vi "PicoScopeospaExampleBlock.vi"() -> ()   [LabVIEW 2010]
uses:
  shared/PicoBuffers.ctl
  <vilib>/Waveform/DWDTOps.llb/DWDT Analog to Digital.vi
  PicoScopepsospaLib/PicoScopeospaDigitalChannelSettings.ctl
  PicoScopepsospaLib/PicoScopeospaAnalogChannelSettings.ctl
  shared/Acquisition Settings.ctl
  shared/Buffer and Transfer Settings.ctl
panel:
  in  "timeIntervalRequested":dbl=2e-10 format="%#6_6p"
  in  "Write ChA to TDMS":bool
  in  "Channels":T1={"Channel A Settings "={"Enabled"=TRUE, "Coupling"=1, "Range"=8, "Analogue Offset"=0.0, "BandWidth"=0, "PROBE_RANGE_INFO"=1}, "Channel B Settings "={"Enabled"=FALSE, "Coupling"=1, "Range"=8, "Analogue Offset"=0.0, "BandWidth"=0, "PROBE_RANGE_INFO"=1}, "Channel C Settings "={"Enabled"=FALSE, "Coupling"=1, "Range"=8, "Analogue Offset"=0.0, "BandWidth"=0, "PROBE_RANGE_INFO"=1}, "Channel D Settings "={"Enabled"=FALSE, "Coupling"=1, "Range"=8, "Analogue Offset"=0.0, "BandWidth"=0, "PROBE_RANGE_INFO"=1}, "Channel E Settings "={"Enabled"=FALSE, "Coupling"=50, "Range"=5, "Analogue Offset"=0.0, "BandWidth"=0, "PROBE_RANGE_INFO"=0}, "Channel F Settings "={"Enabled"=FALSE, "Coupling"=50, "Range"=5, "Analogue Offset"=0.0, "BandWidth"=0, "PROBE_RANGE_INFO"=0}, "Channel G Settings "={"Enabled"=FALSE, "Coupling"=50, "Range"=5, "Analogue Offset"=0.0, "BandWidth"=0, "PROBE_RANGE_INFO"=0}, "Channel H Settings "={"Enabled"=FALSE, "Coupling"=50, "Range"=5, "Analogue Offset"=0.0, "BandWidth"=0, "PROBE_RANGE_INFO"=0}} {"Channel H Settings"."PROBE_RANGE_INFO" items=["PROBE_NONE_NV"=0, "X1_PROBE_NV"=1, "X10_PROBE_NV"=10]; "Channel H Settings"."BandWidth" items=["Full"=0, "100kHz"=100000, "20kHz"=200000, "1MHz"=1000000, "20MHz"=20000000, "25MHz"=25000000, "50MHz"=50000000, "200MHz"=200000000, "250MHz"=250000000, "500MHz"=500000000]; "Channel H Settings"."Range" items=["10mV"=0, "20mV"=1, "50mV"=2, "100mV"=3, "200mV"=4, "500mV"=5, "1V"=6, "2V"=7, "5V"=8, "10V"=9, "20V"=10, "50V"=11, "100V"=12, "200V"=13, "x10_Probe_100mV"=32, "x10_Probe_200mV"=33, "x10_Probe_500mV"=34, "x10_Probe_1V"=35, "x10_Probe_2V"=36, "x10_Probe_5V"=37, "x10_Probe_10V"=38, "x10_Probe_20V"=39, "x10_Probe_50V"=40, "x10_Probe_100V"=41, "x10_Probe_200V"=42, "x10_Probe_500V"=43, "CURRENT_CLAMP_60A_2A"=10500, "CURRENT_CLAMP_60A_5A"=10501, "CURRENT_CLAMP_60A_10A"=10502, "CURRENT_CLAMP_60A_20A"=10503, "CURRENT_CLAMP_60A_50A"=10504, "CURRENT_CLAMP_60A_60A"=10505, "CURRENT_CLAMP_60A_V2_0_5A"=10600, "CURRENT_CLAMP_60A_V2_1A"=10601, "CURRENT_CLAMP_60A_V2_2A"=10602, "CURRENT_CLAMP_60A_V2_5A"=10603, "CURRENT_CLAMP_60A_V2_10A"=10604, "CURRENT_CLAMP_60A_V2_20A"=10605, "CURRENT_CLAMP_60A_V2_50A"=10606, "CURRENT_CLAMP_60A_V2_60A"=10607, "RESISTANCE_LEAD_NEG5_TO_20OHM"=7000, "RESISTANCE_LEAD_NEG50_TO_200OHM"=7001, "RESISTANCE_LEAD_NEG500_TO_2KOHM"=7002, "RESISTANCE_LEAD_NEG5K_TO_20KOHM"=7003, "RESISTANCE_LEAD_NEG50K_TO_LEAD_200KOHM"=7004, "RESISTANCE_LEAD_NEG500K_TO_LEAD_2MOHM"=7005, "RESISTANCE_LEAD_DIODE_TEST"=7006, "HT_NEG3_TO_5KV"=8950, "HT_NEG3_TO_10KV"=8951, "HT_NEG5_TO_20KV"=8952, "HT_NEG5_TO_50KV"=8953, "HT_NEG5_TO_100KV"=8954, "HT_NEG3_TO_5KV_INVERTED"=8955, "HT_NEG3_TO_10KV_INVERTED"=8956, "HT_NEG5_TO_20KV_INVERTED"=8957, "HT_NEG5_TO_50KV_INVERTED"=8958, "HT_NEG5_TO_100KV_INVERTED"=8959, "TEMPERATURE_NEG50_TO_150DEGC"=9000, "PRESSURE_SENSOR_-100k-150k_PASCALS"=9100, "PRESSURE_SENSOR_-100k_TO_400k_PASCALS"=9101, "PRESSURE_SENSOR_-200k_TO_800k_PASCALS"=9102, "PRESSURE_SENSOR_-400k_TO_1600k_PASCALS"=9103, "PRESSURE_SENSOR_-400k_TO_3400k_PASCALS"=9104, "PRESSURE_SENSOR_-150k_TO_1350k_PASCALS"=9105]; "Channel H Settings"."Coupling" items=["AC"=0, "DC 1M Ohm"=1, "DC 50 Ohm"=50]; "Channel G Settings"."PROBE_RANGE_INFO" items=["PROBE_NONE_NV"=0, "X1_PROBE_NV"=1, "X10_PROBE_NV"=10]; "Channel G Settings"."BandWidth" items=["Full"=0, "100kHz"=100000, "20kHz"=200000, "1MHz"=1000000, "20MHz"=20000000, "25MHz"=25000000, "50MHz"=50000000, "200MHz"=200000000, "250MHz"=250000000, "500MHz"=500000000]; "Channel G Settings"."Range" items=["10mV"=0, "20mV"=1, "50mV"=2, "100mV"=3, "200mV"=4, "500mV"=5, "1V"=6, "2V"=7, "5V"=8, "10V"=9, "20V"=10, "50V"=11, "100V"=12, "200V"=13, "x10_Probe_100mV"=32, "x10_Probe_200mV"=33, "x10_Probe_500mV"=34, "x10_Probe_1V"=35, "x10_Probe_2V"=36, "x10_Probe_5V"=37, "x10_Probe_10V"=38, "x10_Probe_20V"=39, "x10_Probe_50V"=40, "x10_Probe_100V"=41, "x10_Probe_200V"=42, "x10_Probe_500V"=43, "CURRENT_CLAMP_60A_2A"=10500, "CURRENT_CLAMP_60A_5A"=10501, "CURRENT_CLAMP_60A_10A"=10502, "CURRENT_CLAMP_60A_20A"=10503, "CURRENT_CLAMP_60A_50A"=10504, "CURRENT_CLAMP_60A_60A"=10505, "CURRENT_CLAMP_60A_V2_0_5A"=10600, "CURRENT_CLAMP_60A_V2_1A"=10601, "CURRENT_CLAMP_60A_V2_2A"=10602, "CURRENT_CLAMP_60A_V2_5A"=10603, "CURRENT_CLAMP_60A_V2_10A"=10604, "CURRENT_CLAMP_60A_V2_20A"=10605, "CURRENT_CLAMP_60A_V2_50A"=10606, "CURRENT_CLAMP_60A_V2_60A"=10607, "RESISTANCE_LEAD_NEG5_TO_20OHM"=7000, "RESISTANCE_LEAD_NEG50_TO_200OHM"=7001, "RESISTANCE_LEAD_NEG500_TO_2KOHM"=7002, "RESISTANCE_LEAD_NEG5K_TO_20KOHM"=7003, "RESISTANCE_LEAD_NEG50K_TO_LEAD_200KOHM"=7004, "RESISTANCE_LEAD_NEG500K_TO_LEAD_2MOHM"=7005, "RESISTANCE_LEAD_DIODE_TEST"=7006, "HT_NEG3_TO_5KV"=8950, "HT_NEG3_TO_10KV"=8951, "HT_NEG5_TO_20KV"=8952, "HT_NEG5_TO_50KV"=8953, "HT_NEG5_TO_100KV"=8954, "HT_NEG3_TO_5KV_INVERTED"=8955, "HT_NEG3_TO_10KV_INVERTED"=8956, "HT_NEG5_TO_20KV_INVERTED"=8957, "HT_NEG5_TO_50KV_INVERTED"=8958, "HT_NEG5_TO_100KV_INVERTED"=8959, "TEMPERATURE_NEG50_TO_150DEGC"=9000, "PRESSURE_SENSOR_-100k-150k_PASCALS"=9100, "PRESSURE_SENSOR_-100k_TO_400k_PASCALS"=9101, "PRESSURE_SENSOR_-200k_TO_800k_PASCALS"=9102, "PRESSURE_SENSOR_-400k_TO_1600k_PASCALS"=9103, "PRESSURE_SENSOR_-400k_TO_3400k_PASCALS"=9104, "PRESSURE_SENSOR_-150k_TO_1350k_PASCALS"=9105]; "Channel G Settings"."Coupling" items=["AC"=0, "DC 1M Ohm"=1, "DC 50 Ohm"=50]; "Channel F Settings"."PROBE_RANGE_INFO" items=["PROBE_NONE_NV"=0, "X1_PROBE_NV"=1, "X10_PROBE_NV"=10]; "Channel F Settings"."BandWidth" items=["Full"=0, "100kHz"=100000, "20kHz"=200000, "1MHz"=1000000, "20MHz"=20000000, "25MHz"=25000000, "50MHz"=50000000, "200MHz"=200000000, "250MHz"=250000000, "500MHz"=500000000]; "Channel F Settings"."Range" items=["10mV"=0, "20mV"=1, "50mV"=2, "100mV"=3, "200mV"=4, "500mV"=5, "1V"=6, "2V"=7, "5V"=8, "10V"=9, "20V"=10, "50V"=11, "100V"=12, "200V"=13, "x10_Probe_100mV"=32, "x10_Probe_200mV"=33, "x10_Probe_500mV"=34, "x10_Probe_1V"=35, "x10_Probe_2V"=36, "x10_Probe_5V"=37, "x10_Probe_10V"=38, "x10_Probe_20V"=39, "x10_Probe_50V"=40, "x10_Probe_100V"=41, "x10_Probe_200V"=42, "x10_Probe_500V"=43, "CURRENT_CLAMP_60A_2A"=10500, "CURRENT_CLAMP_60A_5A"=10501, "CURRENT_CLAMP_60A_10A"=10502, "CURRENT_CLAMP_60A_20A"=10503, "CURRENT_CLAMP_60A_50A"=10504, "CURRENT_CLAMP_60A_60A"=10505, "CURRENT_CLAMP_60A_V2_0_5A"=10600, "CURRENT_CLAMP_60A_V2_1A"=10601, "CURRENT_CLAMP_60A_V2_2A"=10602, "CURRENT_CLAMP_60A_V2_5A"=10603, "CURRENT_CLAMP_60A_V2_10A"=10604, "CURRENT_CLAMP_60A_V2_20A"=10605, "CURRENT_CLAMP_60A_V2_50A"=10606, "CURRENT_CLAMP_60A_V2_60A"=10607, "RESISTANCE_LEAD_NEG5_TO_20OHM"=7000, "RESISTANCE_LEAD_NEG50_TO_200OHM"=7001, "RESISTANCE_LEAD_NEG500_TO_2KOHM"=7002, "RESISTANCE_LEAD_NEG5K_TO_20KOHM"=7003, "RESISTANCE_LEAD_NEG50K_TO_LEAD_200KOHM"=7004, "RESISTANCE_LEAD_NEG500K_TO_LEAD_2MOHM"=7005, "RESISTANCE_LEAD_DIODE_TEST"=7006, "HT_NEG3_TO_5KV"=8950, "HT_NEG3_TO_10KV"=8951, "HT_NEG5_TO_20KV"=8952, "HT_NEG5_TO_50KV"=8953, "HT_NEG5_TO_100KV"=8954, "HT_NEG3_TO_5KV_INVERTED"=8955, "HT_NEG3_TO_10KV_INVERTED"=8956, "HT_NEG5_TO_20KV_INVERTED"=8957, "HT_NEG5_TO_50KV_INVERTED"=8958, "HT_NEG5_TO_100KV_INVERTED"=8959, "TEMPERATURE_NEG50_TO_150DEGC"=9000, "PRESSURE_SENSOR_-100k-150k_PASCALS"=9100, "PRESSURE_SENSOR_-100k_TO_400k_PASCALS"=9101, "PRESSURE_SENSOR_-200k_TO_800k_PASCALS"=9102, "PRESSURE_SENSOR_-400k_TO_1600k_PASCALS"=9103, "PRESSURE_SENSOR_-400k_TO_3400k_PASCALS"=9104, "PRESSURE_SENSOR_-150k_TO_1350k_PASCALS"=9105]; "Channel F Settings"."Coupling" items=["AC"=0, "DC 1M Ohm"=1, "DC 50 Ohm"=50]; "Channel E Settings"."PROBE_RANGE_INFO" items=["PROBE_NONE_NV"=0, "X1_PROBE_NV"=1, "X10_PROBE_NV"=10]; "Channel E Settings"."BandWidth" items=["Full"=0, "100kHz"=100000, "20kHz"=200000, "1MHz"=1000000, "20MHz"=20000000, "25MHz"=25000000, "50MHz"=50000000, "200MHz"=200000000, "250MHz"=250000000, "500MHz"=500000000]; "Channel E Settings"."Range" items=["10mV"=0, "20mV"=1, "50mV"=2, "100mV"=3, "200mV"=4, "500mV"=5, "1V"=6, "2V"=7, "5V"=8, "10V"=9, "20V"=10, "50V"=11, "100V"=12, "200V"=13, "x10_Probe_100mV"=32, "x10_Probe_200mV"=33, "x10_Probe_500mV"=34, "x10_Probe_1V"=35, "x10_Probe_2V"=36, "x10_Probe_5V"=37, "x10_Probe_10V"=38, "x10_Probe_20V"=39, "x10_Probe_50V"=40, "x10_Probe_100V"=41, "x10_Probe_200V"=42, "x10_Probe_500V"=43, "CURRENT_CLAMP_60A_2A"=10500, "CURRENT_CLAMP_60A_5A"=10501, "CURRENT_CLAMP_60A_10A"=10502, "CURRENT_CLAMP_60A_20A"=10503, "CURRENT_CLAMP_60A_50A"=10504, "CURRENT_CLAMP_60A_60A"=10505, "CURRENT_CLAMP_60A_V2_0_5A"=10600, "CURRENT_CLAMP_60A_V2_1A"=10601, "CURRENT_CLAMP_60A_V2_2A"=10602, "CURRENT_CLAMP_60A_V2_5A"=10603, "CURRENT_CLAMP_60A_V2_10A"=10604, "CURRENT_CLAMP_60A_V2_20A"=10605, "CURRENT_CLAMP_60A_V2_50A"=10606, "CURRENT_CLAMP_60A_V2_60A"=10607, "RESISTANCE_LEAD_NEG5_TO_20OHM"=7000, "RESISTANCE_LEAD_NEG50_TO_200OHM"=7001, "RESISTANCE_LEAD_NEG500_TO_2KOHM"=7002, "RESISTANCE_LEAD_NEG5K_TO_20KOHM"=7003, "RESISTANCE_LEAD_NEG50K_TO_LEAD_200KOHM"=7004, "RESISTANCE_LEAD_NEG500K_TO_LEAD_2MOHM"=7005, "RESISTANCE_LEAD_DIODE_TEST"=7006, "HT_NEG3_TO_5KV"=8950, "HT_NEG3_TO_10KV"=8951, "HT_NEG5_TO_20KV"=8952, "HT_NEG5_TO_50KV"=8953, "HT_NEG5_TO_100KV"=8954, "HT_NEG3_TO_5KV_INVERTED"=8955, "HT_NEG3_TO_10KV_INVERTED"=8956, "HT_NEG5_TO_20KV_INVERTED"=8957, "HT_NEG5_TO_50KV_INVERTED"=8958, "HT_NEG5_TO_100KV_INVERTED"=8959, "TEMPERATURE_NEG50_TO_150DEGC"=9000, "PRESSURE_SENSOR_-100k-150k_PASCALS"=9100, "PRESSURE_SENSOR_-100k_TO_400k_PASCALS"=9101, "PRESSURE_SENSOR_-200k_TO_800k_PASCALS"=9102, "PRESSURE_SENSOR_-400k_TO_1600k_PASCALS"=9103, "PRESSURE_SENSOR_-400k_TO_3400k_PASCALS"=9104, "PRESSURE_SENSOR_-150k_TO_1350k_PASCALS"=9105]; "Channel E Settings"."Coupling" items=["AC"=0, "DC 1M Ohm"=1, "DC 50 Ohm"=50]; "Channel D Settings"."BandWidth" items=["Full"=0, "100kHz"=100000, "20kHz"=200000, "1MHz"=1000000, "20MHz"=20000000, "25MHz"=25000000, "50MHz"=50000000, "100MHz"=100000000, "200MHz"=200000000, "250MHz"=250000000, "350MHz"=350000000, "500MHz"=500000000]; "Channel D Settings"."PROBE_RANGE_INFO" items=["PROBE_NONE_NV"=0, "X1_PROBE_NV"=1, "X10_PROBE_NV"=10]; "Channel D Settings"."Range" items=["10mV", "20mV", "50mV", "100mV", "200mV", "500mV", "1V", "2V", "5V", "10V", "20V", "50V", "100V", "200V"]; "Channel D Settings"."Coupling" items=["AC"=0, "DC 1M Ohm"=1, "DC 50 Ohm"=50]; "Channel C Settings"."BandWidth" items=["Full"=0, "100kHz"=100000, "20kHz"=200000, "1MHz"=1000000, "20MHz"=20000000, "25MHz"=25000000, "50MHz"=50000000, "100MHz"=100000000, "200MHz"=200000000, "250MHz"=250000000, "350MHz"=350000000, "500MHz"=500000000]; "Channel C Settings"."PROBE_RANGE_INFO" items=["PROBE_NONE_NV"=0, "X1_PROBE_NV"=1, "X10_PROBE_NV"=10]; "Channel C Settings"."Range" items=["10mV", "20mV", "50mV", "100mV", "200mV", "500mV", "1V", "2V", "5V", "10V", "20V", "50V", "100V", "200V"]; "Channel C Settings"."Coupling" items=["AC"=0, "DC 1M Ohm"=1, "DC 50 Ohm"=50]; "Channel B Settings"."BandWidth" items=["Full"=0, "100kHz"=100000, "20kHz"=200000, "1MHz"=1000000, "20MHz"=20000000, "25MHz"=25000000, "50MHz"=50000000, "100MHz"=100000000, "200MHz"=200000000, "250MHz"=250000000, "350MHz"=350000000, "500MHz"=500000000]; "Channel B Settings"."PROBE_RANGE_INFO" items=["PROBE_NONE_NV"=0, "X1_PROBE_NV"=1, "X10_PROBE_NV"=10]; "Channel B Settings"."Range" items=["10mV", "20mV", "50mV", "100mV", "200mV", "500mV", "1V", "2V", "5V", "10V", "20V", "50V", "100V", "200V"]; "Channel B Settings"."Coupling" items=["AC"=0, "DC 1M Ohm"=1, "DC 50 Ohm"=50]; "Channel A Settings"."PROBE_RANGE_INFO" items=["PROBE_NONE_NV"=0, "X1_PROBE_NV"=1, "X10_PROBE_NV"=10]; "Channel A Settings"."Range" items=["10mV", "20mV", "50mV", "100mV", "200mV", "500mV", "1V", "2V", "5V", "10V", "20V", "50V", "100V", "200V"]; "Channel A Settings"."BandWidth" items=["Full"=0, "100kHz"=100000, "20kHz"=200000, "1MHz"=1000000, "20MHz"=20000000, "25MHz"=25000000, "50MHz"=50000000, "100MHz"=100000000, "200MHz"=200000000, "250MHz"=250000000, "350MHz"=350000000, "500MHz"=500000000]; "Channel A Settings"."Coupling" items=["AC"=0, "DC 1M Ohm"=1, "DC 50 Ohm"=50]}
  out "error out":errorcluster
  in  "Data file":path=path "PicoScopeospaExampleBlock ChA Data"
  out "overflow":i16 format="%010b"
  in  "Apply Settings":bool
  in  "Digital Channels":T2={"Port 0 Settings "={"Enabled"=FALSE, "Threshold Level (Volts)"=1.0}, "Port 1 Settings"={"Enabled"=FALSE, "Threshold Level (Volts)"=1.0}} {"Port 1 Settings"."Threshold Level (Volts)" format="%#_4p"; "Port 0 Settings"."Threshold Level (Volts)" format="%#_4p"}
  in  "Trigger Settings":T3={"Trigger Enabled"=FALSE, "Trigger Threshold (Volts)"=0.0, "Trigger Direction"=2, "Trigger Delay (samples)"=0, "Auto Trigger Time (us)"=1000000, "Trigger Source"=0} {"Trigger Source" items=["Channel A"=0, "Channel B"=1, "Channel C"=2, "Channel D"=3, "Channel E"=4, "Channel F"=5, "Channel G"=6, "Channel H"=7, "Port 0"=128, "Port 1"=129, "Trigger AUX"=1001]; "Auto Trigger Time (us)" format="%.4p"; "Trigger Direction" items=["Above", "Below", "Rising", "Falling", "Rising or Falling"]; "Trigger Threshold (Volts)" format="%#_6p"}
  in  "Buffer and Transfer Settings":T4={"startIndex"=0, "Samples"=10000000, "Down Sample Ratio"=16, "Down-Sample Mode"=2} {"Down-Sample Mode" items=["RAW none"=2147483648, "None"=0, "Aggregate"=1, "Decimate"=2, "Average"=4]; "Down Sample Ratio" step=1; "Samples" format="%_6p"}
  in  "Acquisition Settings":T5={"preTriggerSamples"=0, "postTriggerSamples"=100000000, "timebase"=2} {"postTriggerSamples" format="%_6p"; "preTriggerSamples" format="%_6p"}
  out "Properties Panel":T6 {"Max Total Capture Time Available (sec)" format="%.3p"; "Sample Frequency" format="%.6p"; "Sample Rate" format="%.3p"; "Max Samples Available" format="%_6p"; "Total Capture Time (sec)" format="%.3p"}
  out "Port 0":digitalwaveform(graph)={"t0"=timestamp(0 s since 1904-01-01), "dt"=4e-09, "Y"={"transitions"=[], "data"=[]}}
  in  "stop":bool
  out "Analog Channels":cluster{i32, dbl, "Data":dbl[]}[](graph)
  out "Device Info":T7={"PICO_DRIVER_VERSION"="", "PICO_USB_VERSION"="", "PICO_HARDWARE_VERSION"="", "PICO_VARIANT_INFO"="", "PICO_BATCH_AND_SERIAL"="", "PICO_CAL_DATE"="", "PICO_KERNEL_VERSION"="", "PICO_DIGITAL_HARDWARE_VERSION"="", "PICO_ANALOGUE_HARDWARE_VERSION"="", "PICO_FIRMWARE_VERSION_1"="", "PICO_FIRMWARE_VERSION_2"="", "PICO_IPP_VERSION"="", "PICO_DRIVER_PATH"="", "PICO_FIRMWARE_VERSION_3"="", "PICO_FRONT_PANEL_FIRMWARE_VERSION"="", "Number of Channels"=4, "MSO"=FALSE}
  out "Pico psospa Units":string
  in  "Resolution":u32(ring) items=["8-bit"=0, "12-bit"=1, "14-bit"=2, "15-bit"=3, "16-bit"=4, "10-bit"=10]
  in  "Serial Number":string
  in  "Use Serial Number":bool
  in  "error in (no error)":errorcluster
  # "D8-D15"
  # "DO-D7"
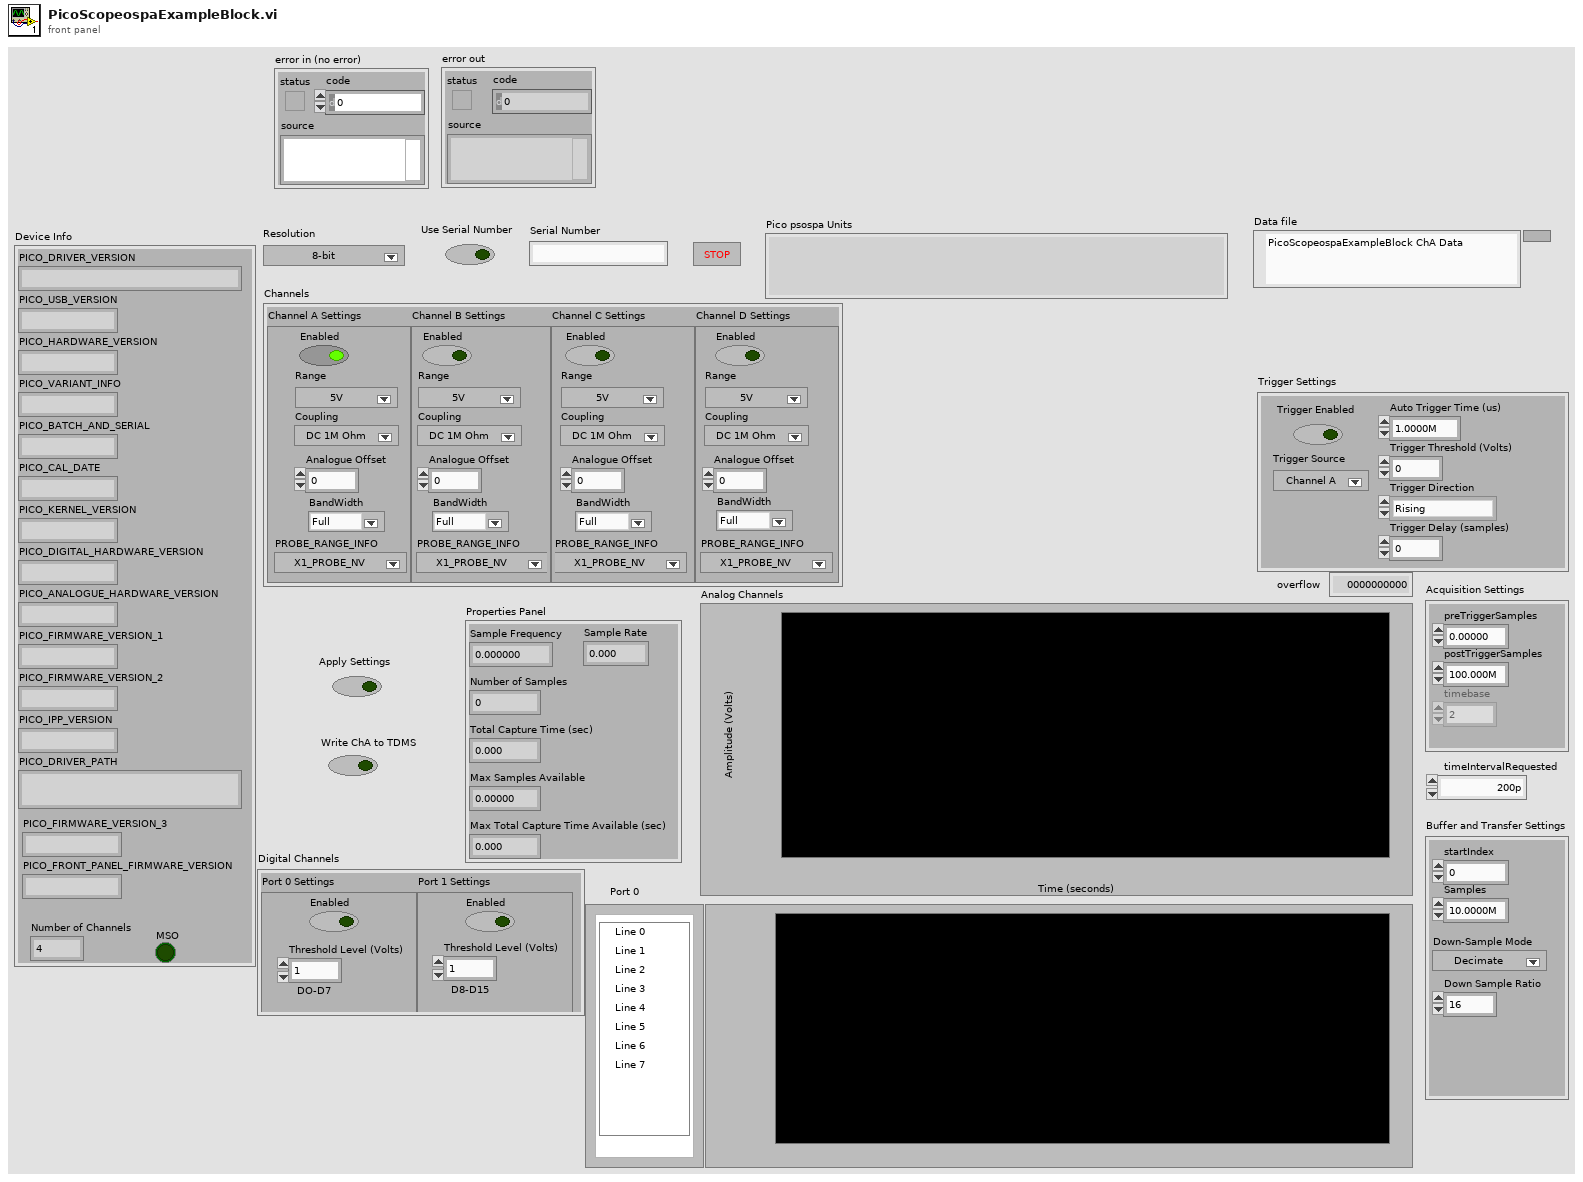
[diagram p1: front panel]
types:
  T1 = typedef "PicoScopeospaAnalogChannelSettings.ctl" = cluster{"Channel A Settings ":cluster{"Enabled":bool, "Coupling":i16, "Range":u16, "Analogue Offset":dbl, "BandWidth":u32, "PROBE_RANGE_INFO":u32}, "Channel B Settings ":cluster{"Enabled":bool, "Coupling":i16, "Range":u16, "Analogue Offset":dbl, "BandWidth":u32, "PROBE_RANGE_INFO":u32}, "Channel C Settings ":cluster{"Enabled":bool, "Coupling":i16, "Range":u16, "Analogue Offset":dbl, "BandWidth":u32, "PROBE_RANGE_INFO":u32}, "Channel D Settings ":cluster{"Enabled":bool, "Coupling":i16, "Range":u16, "Analogue Offset":dbl, "BandWidth":u32, "PROBE_RANGE_INFO":u32}, "Channel E Settings ":cluster{"Enabled":bool, "Coupling":i16, "Range":u16, "Analogue Offset":dbl, "BandWidth":u32, "PROBE_RANGE_INFO":u32}, "Channel F Settings ":cluster{"Enabled":bool, "Coupling":i16, "Range":u16, "Analogue Offset":dbl, "BandWidth":u32, "PROBE_RANGE_INFO":u32}, "Channel G Settings ":cluster{"Enabled":bool, "Coupling":i16, "Range":u16, "Analogue Offset":dbl, "BandWidth":u32, "PROBE_RANGE_INFO":u32}, "Channel H Settings ":cluster{"Enabled":bool, "Coupling":i16, "Range":u16, "Analogue Offset":dbl, "BandWidth":u32, "PROBE_RANGE_INFO":u32}}
  T2 = typedef "PicoScopeospaDigitalChannelSettings.ctl" = cluster{"Port 0 Settings ":cluster{"Enabled":bool, "Threshold Level (Volts)":dbl}, "Port 1 Settings":cluster{"Enabled":bool, "Threshold Level (Volts)":dbl}}
  T3 = cluster{"Trigger Enabled":bool, "Trigger Threshold (Volts)":dbl, "Trigger Direction":u16, "Trigger Delay (samples)":u64, "Auto Trigger Time (us)":u32, "Trigger Source":u32}
  T4 = typedef "Buffer and Transfer Settings.ctl" = cluster{"startIndex":u64, "Samples":u64, "Down Sample Ratio":u64, "Down-Sample Mode":u32}
  T5 = typedef "Acquisition Settings.ctl" = cluster{"preTriggerSamples":u64, "postTriggerSamples":u64, "timebase":u32}
  T6 = cluster{"Sample Frequency":dbl, "Sample Rate":dbl, "Max Samples Available":u64, "Number of Samples":u64, "Total Capture Time (sec) ":dbl, "Max Total Capture Time Available (sec)":dbl}
  T7 = cluster{"PICO_DRIVER_VERSION":string, "PICO_USB_VERSION":string, "PICO_HARDWARE_VERSION":string, "PICO_VARIANT_INFO":string, "PICO_BATCH_AND_SERIAL":string, "PICO_CAL_DATE":string, "PICO_KERNEL_VERSION":string, "PICO_DIGITAL_HARDWARE_VERSION":string, "PICO_ANALOGUE_HARDWARE_VERSION":string, "PICO_FIRMWARE_VERSION_1":string, "PICO_FIRMWARE_VERSION_2":string, "PICO_IPP_VERSION":string, "PICO_DRIVER_PATH":string, "PICO_FIRMWARE_VERSION_3":string, "PICO_FRONT_PANEL_FIRMWARE_VERSION":string, "Number of Channels":i16, "MSO":bool}
  T8 = enum16{"open", "open or create", "create or replace", "create", "open (read-only)"}
  T9 = typedef "PicoBuffers.ctl" = cluster{"Max Buffer Pointers":u64[][][], "Min Buffer Pointers":u64[][][], "StreamingDataInfo":cluster{"Channel":u32, "Down-Sample Mode":u32, "PICO_DATA_TYPE":enum32{"PICO_INT8_T", "PICO_INT16_T", "PICO_INT32_T", "PICO_UINT32_T", "PICO_INT64_T", ""}, "Samples":i32, "bufferIndex":u64, "startIndex":i32, "overflow":i16}[][]}
  T10 = cluster{"Channel A Buffer":i16[], "Channel B Buffer":i16[], "Channel C Buffer":i16[], "Channel D Buffer":i16[], "Channel E Buffer":i16[], "Channel F Buffer":i16[], "Channel G Buffer":i16[], "Channel H Buffer":i16[], "Port 0 Buffer":i16[], "Port 1 Buffer":i16[]}[]
  T11 = cluster{"Channel A Buffer":i16[], "Channel B Buffer":i16[], "Channel C Buffer":i16[], "Channel D Buffer":i16[], "Channel E Buffer":i16[], "Channel F Buffer":i16[], "Channel G Buffer":i16[], "Channel H Buffer":i16[], "Port 0 Buffer":i16[], "Port 1 Buffer":i16[]}
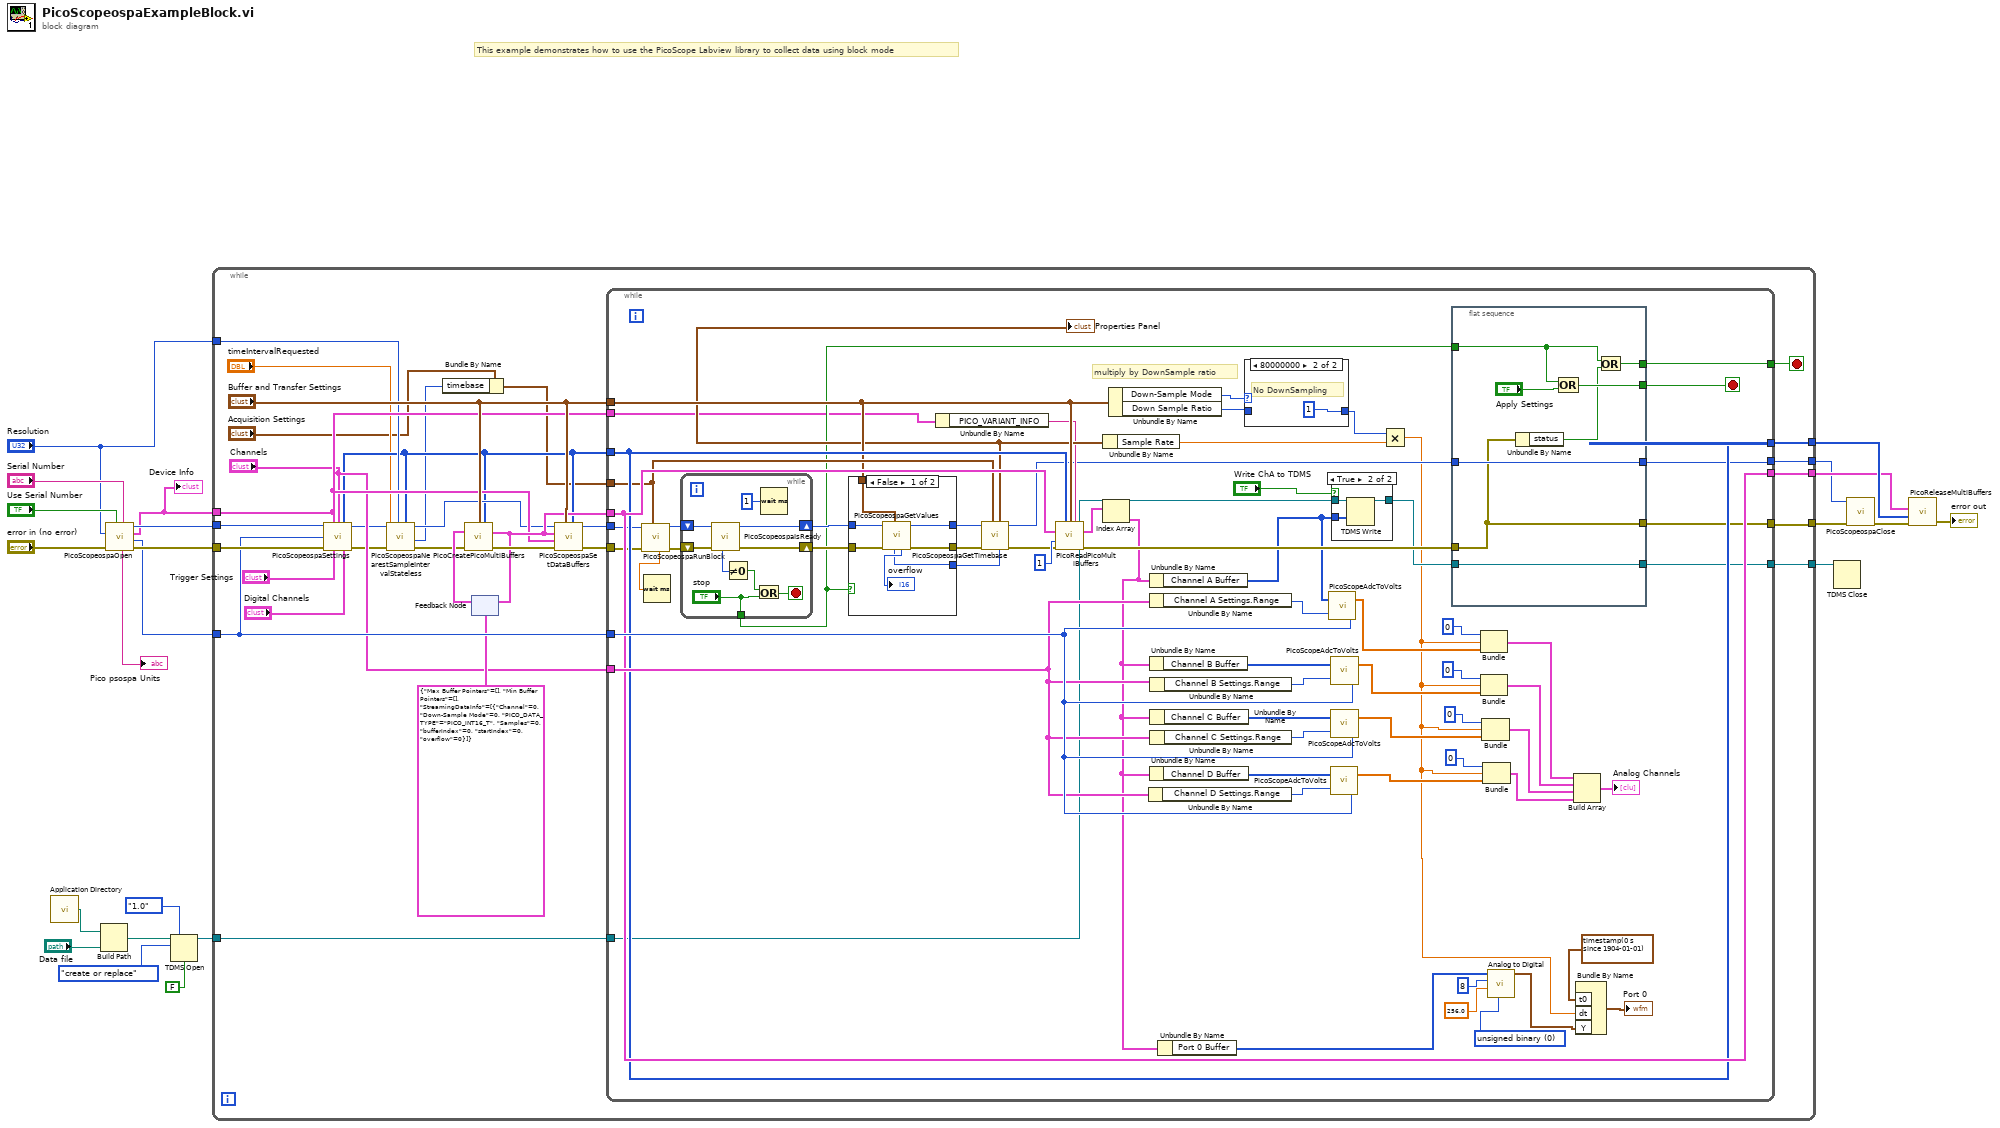
[diagram p0: block diagram]
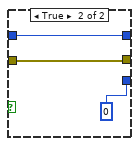
[diagram p3: hidden frame]
diagram:
  # "This example demonstrates how to use the PicoScope Labview library to collect data using block mode"
  n1 = call <vilib>:"Application Directory.vi"() -> ("Application Directory"=w5:path)
  n2 = Build Path(base path=w5, name or relative path="Data file") -> (appended path=w6:path)
  n3 = call "PicoScopeospaOpen.vi"("Serial Number"="Serial Number", "Use Serial Number"="Use Serial Number", "error in (no error)"="error in (no error)", "Resolution"="Resolution") -> ("error out"=w19:errorcluster, "Max ADC value"=w17:i16, "Device Info"=w16:T7, "handle out"=w20:i16, "Pico psospa Units"=→"Pico psospa Units":string)  [unwired: 2 in, 1 out]
  "Device Info" <- w16
  n4 = TDMS Open(6:FALSE ("disable buffering? (T)"), 7:enum16{"1.0", "2.0"}."1.0" ("file format version (2.0)"), 10:T8."create or replace" ("operation (0:open)"), 11:w6) -> (3:w3:refnum<k34>)  [unwired: 2 in, 1 out]
  n5 = while {
    tunnel: w16 -> [w35]
    tunnel: w17 -> [w52]
    tunnel: w20 -> [w54]
    tunnel: [w47] -> w12
    tunnel: w19 -> [w53]
    tunnel: [w45] -> w13
    tunnel: [w44] -> w15
    tunnel: [w49] -> w14
    tunnel: [w37] -> w4
    tunnel: w3 -> [w36]
    tunnel: "Resolution" -> [w29]
    stop <- w38 stop-if-true
    n6 = call "PicoScopeospaSettings.vi"("handle in"=w54, "Device Info"=w35, "Channels"="Channels", "Max ADC value"=w52, "error in (no error)"=w53, "Trigger Settings"="Trigger Settings", "Digital Channels"="Digital Channels") -> ("Enabled array"=w28:i16[], "handle out"=w30:i16, "error out"=w33:errorcluster)  [unwired: 6 in]
    n7 = call "PicoScopeospaNearestSampleIntervalStateless.vi"("Enabled array"=w28, "Resolution"=w29, "error in (no error)"=w33, "timeIntervalRequested"="timeIntervalRequested", "handle in"=w30) -> ("error out"=w32:errorcluster, "timebase"=w24:u32, "handle out"=w31:i16)  [unwired: 3 in, 1 out]
    n8 = Bundle By Name(cluster="Acquisition Settings", "timebase"=w24) -> (w25:T5)
    n9 = feedback #1(T9 {"Max Buffer Pointers"=[], "Min Buffer Pointers"=[], "StreamingDataInfo"=[[{"Channel"=0, "Down-Sample Mode"=0, "PICO_DATA_TYPE"=enum."PICO_INT16_T", "Samples"=0, "bufferIndex"=0, "startIndex"=0, "overflow"=0}]]} ("Data Pointers")) -> (w48:T9)
    n10 = call "PicoCreatePicoMultiBuffers.vi"("Buffer and Transfer Settings"="Buffer and Transfer Settings", "enabled array"=w28, "Data Pointers In"=w48, "error in (no error)"=w32) -> ("Data Pointers"=w40:T9, "error out"=w43:errorcluster)  [unwired: 10 in]
    n11 = feedback-in #1(w40) -> ()
    n12 = call "PicoScopeospaSetDataBuffers.vi"("enabled array"=w28, "Buffer and Transfer Settings"="Buffer and Transfer Settings", "error in (no error)"=w43, "Device Info"=w35, "Data Pointers In"=w40, "handle in"=w31) -> ("error out"=w42:errorcluster, "handle out"=w39:i16)  [unwired: 4 in]
    n13 = while {
      tunnel: w52 -> [w121]
      tunnel: w25 -> [w117]
      tunnel: "Channels" -> [w120]
      tunnel: [w72] -> w45
      tunnel: [w119] -> w49
      tunnel: "Buffer and Transfer Settings" -> [w116]
      tunnel: w42 -> [w60]
      tunnel: [w74] -> w47
      tunnel: w39 -> [w59]
      tunnel: w40 -> [w119]
      tunnel: [w118] -> w44
      tunnel: w28 -> [w118]
      tunnel: [w75] -> w38
      tunnel: [w71] -> w37
      tunnel: w36 -> [w69]
      tunnel: w35 -> [w65]
      stop <- w115 stop-if-true
      w94 = u16 0 items=["unsigned binary", "offset binary", "2's complement"] ("data format (offset binary)")
      # "multiply by DownSample ratio"
      n14 = call "PicoScopeospaRunBlock.vi"("Acquisition Settings"=w117, "error in (no error)"=w60, "handle in"=w59) -> ("error out"=w80:errorcluster, "handle out"=w77:i16, "timeIndisposedMs"=w57:dbl)  [unwired: 5 in, 1 out]
      n15 = Wait (ms)(milliseconds to wait=w57) -> ()  [unwired: 1 out]
      n16 = while {
        shift-right: [w151] -> w79
        shift-left: w80 -> [w152]
        shift-right: [w150] -> w78
        shift-left: w77 -> [w149]
        tunnel: ["stop"] -> w76
        stop <- w147 stop-if-true
        n17 = call "PicoScopeospaIsReady.vi"("error in (no error)"=w152, "handle in"=w149) -> ("error out"=w151:errorcluster, "handle out"=w150:i16, "ready"=w148:i16)  [unwired: 7 in]
        n18 = Not Equal To 0?(x=w148) -> (x != 0?=w146:bool)
        n19 = Or(x=w146, y="stop") -> (x .or. y?=w147:bool)
        n20 = Wait (ms)(milliseconds to wait=u32 1) -> ()  [unwired: 1 out]
      }
      n21 = case shown="False" w76 {
        tunnel: w79 -> [w140 w143]
        tunnel: [w139 w143] -> w63
        tunnel: [w138 w142] -> w58
        tunnel: w78 -> [w137 w142]
        tunnel: w116 -> [w136 _]
        tunnel: [w134 u64 0 ("noOfSamples")] -> w62
        frame False {
          n22 = call "PicoScopeospaGetValues.vi"("Buffer and Transfer Settings"=w136, "error in (no error)"=w140, "handle in"=w137) -> ("error out"=w139:errorcluster, "handle out"=w138:i16, "overflow"=→"overflow":i16, "noOfSamples"=w134:u64)  [unwired: 5 in]
        }
        frame True {
        }
      }
      n23 = Unbundle By Name(w65) -> ("PICO_VARIANT_INFO"=w66:string)
      n24 = call "PicoScopeospaGetTimebase.vi"("Number of Samples"=w62, "Acquisition Settings"=w117, "error in (no error)"=w63, "handle in"=w58) -> ("error out"=w61:errorcluster, "handle out"=w64:i16, "Properties Panel"=w82:T6)  [unwired: 5 in]
      "Properties Panel" <- w82
      n25 = call "PicoReadPicoMultiBuffers.vi"("enabled array"=w118, "Buffer and Transfer Settings"=w116, "Variant"=w66, "Data Pointers"=w119, "No of Buffers"=1, "error in (no error)"=w61) -> ("MultiBuffers (Max or non-aggregated)"=w87:T10, "error out"=w73:errorcluster)  [unwired: 7 in, 1 out]
      n26 = Index Array(array=w87) -> (element=w68:T11)  [unwired: 1 in]
      n27 = Unbundle By Name(w82) -> ("Sample Rate"=w85:dbl)
      n28 = Unbundle By Name(w116) -> ("Down-Sample Mode"=w83:u32, "Down Sample Ratio"=w84:u64)
      n29 = Unbundle By Name(w120) -> ("Channel D Settings.Range"=w102:u16)
      n30 = Unbundle By Name(w68) -> ("Channel A Buffer"=w67:i16[])
      n31 = Unbundle By Name(w120) -> ("Channel A Settings.Range"=w113:u16)
      n32 = Unbundle By Name(w68) -> ("Channel B Buffer"=w111:i16[])
      n33 = Unbundle By Name(w68) -> ("Channel D Buffer"=w103:i16[])
      n34 = Unbundle By Name(w120) -> ("Channel B Settings.Range"=w110:u16)
      n35 = Unbundle By Name(w68) -> ("Channel C Buffer"=w105:i16[])
      n36 = Unbundle By Name(w120) -> ("Channel C Settings.Range"=w104:u16)
      n37 = Unbundle By Name(w68) -> ("Port 0 Buffer"=w92:i16[])
      n38 = case shown="80000000" w83 {
        tunnel: [w153 u64 1 ("Down Sample Ratio")] -> w81
        tunnel: w84 -> [w153 _]
        frame Default {
        }
        frame -2147483648 {
          # "No DownSampling"
        }
      }
      n39 = call "PicoScopeAdcToVolts.vi"("Max_adc"=w121, "Range Index"=w113, "Data"=w67) -> ("Data"=w88:dbl[])
      n40 = call "PicoScopeAdcToVolts.vi"("Max_adc"=w121, "Range Index"=w102, "Data"=w103) -> ("Data"=w98:dbl[])
      n41 = call "PicoScopeAdcToVolts.vi"("Max_adc"=w121, "Range Index"=w110, "Data"=w111) -> ("Data"=w109:dbl[])
      n42 = call "PicoScopeAdcToVolts.vi"("Max_adc"=w121, "Range Index"=w104, "Data"=w105) -> ("Data"=w99:dbl[])
      n43 = case shown="True" "Write ChA to TDMS" {
        tunnel: [w122 w125] -> w70
        tunnel: w69 -> [w122 w124]
        tunnel: w67 -> [_ w123]
        frame False {
        }
        frame True {
          n44 = TDMS Write(0:w124, 9:w123) -> (4:w125:refnum<k34>)  [unwired: 4 in, 3 out]
        }
      }
      n45 = Multiply(x=w81, y=w85) -> (x*y=w56:dbl)
      n46 = flat-sequence {
        tunnel: [w133] -> w115
        tunnel: w76 -> [w131]
        tunnel: [w129] -> w75
        tunnel: w64 -> [w128]
        tunnel: [w128] -> w74
        tunnel: w73 -> [w127]
        tunnel: [w127] -> w72
        tunnel: [w126] -> w71
        tunnel: w70 -> [w126]
        frame #0 {
          n47 = Unbundle By Name(w127) -> ("status"=w130:bool)
          n48 = Compound Arithmetic op=OR(w131, "Apply Settings") -> (w133:bool)
          n49 = Or(x=w131, y=w130) -> (x .or. y?=w129:bool)
        }
      }
      n50 = Bundle(0, w56, "Data"=w88) -> (w108:cluster{i32, dbl, "Data":dbl[]})  [unwired: 1 in]
      n51 = Bundle(0, w56, "Data"=w109) -> (w107:cluster{i32, dbl, "Data":dbl[]})  [unwired: 1 in]
      n52 = Bundle(0, w56, "Data"=w99) -> (w97:cluster{i32, dbl, "Data":dbl[]})  [unwired: 1 in]
      n53 = Bundle(0, w56, "Data"=w98) -> (w96:cluster{i32, dbl, "Data":dbl[]})  [unwired: 1 in]
      n54 = call-poly <vilib>:"Analog to Digital.vi"("data format (offset binary)"=w94, "full-scale range (pk-pk)"=256.0, "resolution (16 bit)"=8, "analog waveform"=w92) -> ("digital waveform"=w89:digitalwaveform)  [unwired: 4 in, 3 out]
      n55 = Build Array(w108, w107, w97, w96) -> (→"Analog Channels":cluster{i32, dbl, "Data":dbl[]}[])
      n56 = Bundle By Name("t0"=timestamp(0 s since 1904-01-01), "dt"=w56, "Y"=w89) -> (→"Port 0":digitalwaveform)  [unwired: 1 in]
    }
  }
  n57 = TDMS Close(11:w4) -> ()  [unwired: 1 in, 2 out]
  n58 = call "PicoScopeospaClose.vi"("error in (no error)"=w13, "handle in"=w12) -> ("error out"=w11:errorcluster)  [unwired: 8 in, 1 out]
  n59 = call "PicoReleaseMultiBuffers.vi"("error in (no error)"=w11, "Enabled array"=w15, "Data Pointers"=w14) -> ("error out"=→"error out":errorcluster)  [unwired: 7 in, 1 out]
